vi "Update Path.vi"(8 "Error In":errorcluster, 11 "Measurement specfic paths":T2=enum."Harmonics") -> (0 "Error Out":errorcluster, 3 "Current Paths":T1(array[cluster]))   [LabVIEW 2020, in "PathControl.lvclass"]
uses:
  PathControl.lvclass
  Measurements Specific Paths.ctl
  <vilib>/Utility/xml.llb/Read From XML File(string).vi
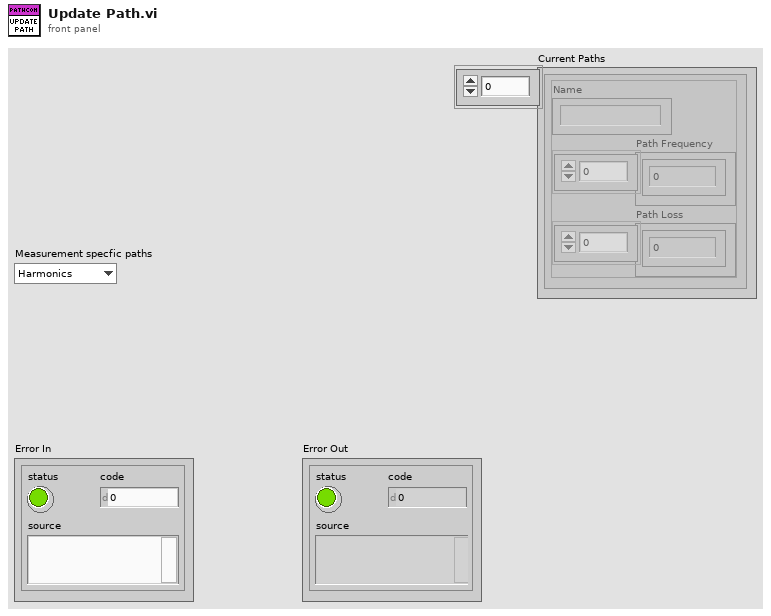
[diagram p1: front panel]
types:
  T1 = cluster{"Name":string, "Path Frequency":dbl[], "Path Loss":dbl[]}[]
  T2 = typedef "PathControl.lvclass/Measurements Specific Paths.ctl" = enum16{"No calibration", "Harmonics", "IMD", "S Parameter", "AM-AM", "MCCW-ACLR", "DC", "LCR", "Power Meter GUI", "RF Power"}
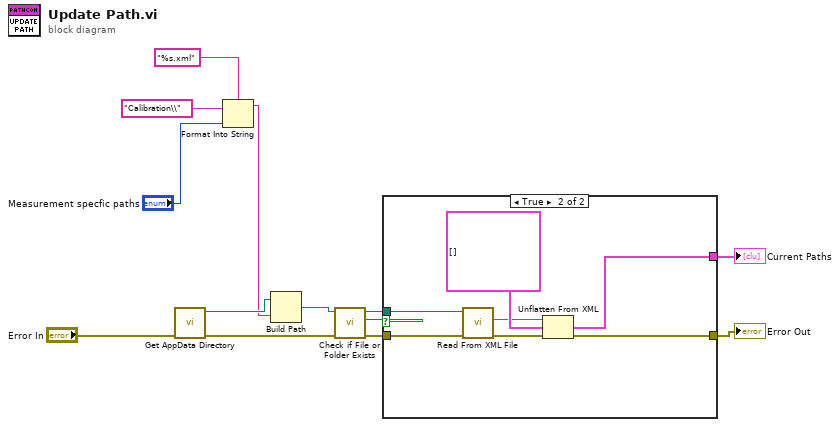
[diagram p0: block diagram]
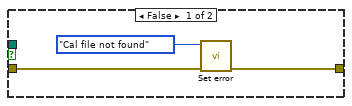
[diagram p2: hidden frame]
diagram:
  n1 = call "Get AppData Directory.vi"("Error In"="Error In") -> ("Error Out"=w6:errorcluster, "Folder path"=w12:path)  [unwired: 8 in, 1 out]
  n2 = Format Into String(format string="%s.xml", initial string="Calibration\\" ("name or relative path"), "Measurement specfic paths") -> (resulting string=w8:string)  [unwired: 1 in, 1 out]
  n3 = Build Path(base path=w12, name or relative path=w8) -> (appended path=w7:path)
  n4 = call <vilib>:"Check if File or Folder Exists.vi"("error in (no error)"=w6, "path"=w7) -> ("error out"=w4:errorcluster, "file or folder exists?"=w5:bool, "dup path"=w3:path)  [unwired: 7 in]
  n5 = case shown="True" w5 {
    tunnel: w4 -> [w16 w19]
    tunnel: w3 -> [_ w20]
    tunnel: [w14 w22] -> w2
    tunnel: [_ w21] -> w1
    frame False {
      n6 = call "Set error.vi"("Error In"=w16, "Errors"=enum16{"Cal file not found"}."Cal file not found") -> ("Error Out"=w14:errorcluster)  [unwired: 9 in]
    }
    frame True {
      n7 = call-poly <vilib>:"Read From XML File.vi"("error in (no error)"=w19, "XML File Path"=w20) -> ("error out"=w18:errorcluster, "XML Elements"=w17:string)  [unwired: 7 in, 1 out]
      n8 = Unflatten From XML(xml string=w17, type=T1 [] ("Current Paths"), error in (no error)=w18) -> (value=w21:T1, error out=w22:errorcluster)
    }
  }
  "Error Out" <- w2
  "Current Paths" <- w1
